vi "Register Assert.vi"(11 "Properties.Assert in":refnum<class "Properties.Assert.lvclass">) -> (3 "Properties.Assert out":refnum<class "Properties.Assert.lvclass">)   [LabVIEW 2013, in "Caraya.lvlib" / "Properties.Assert.lvclass"]
uses:
  Properties.Assert.lvclass
  Test Manager Message Assertion/TestManagerMsg.Assertion.lvclass
  Test Manager Message Assertion/Assert-Data -- cluster.ctl
  Properties.Assert.lvclass/Properties.Assert.ctl
  Properties/Properties.lvclass/Properties.ctl
  Properties/Properties.lvclass
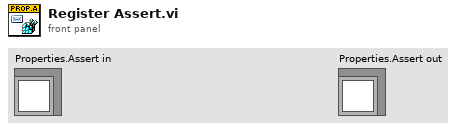
[diagram p1: front panel]
types:
  T1 = typedef "Caraya.lvlib/TestManagerMsg.Assertion.lvclass/Assert-Data -- cluster.ctl" = cluster{"Label":string, "Asserted":bool, "call-chain":string[], "upstream-error":errorcluster, "timestamp":timestamp, "Execution time (s)":dbl}
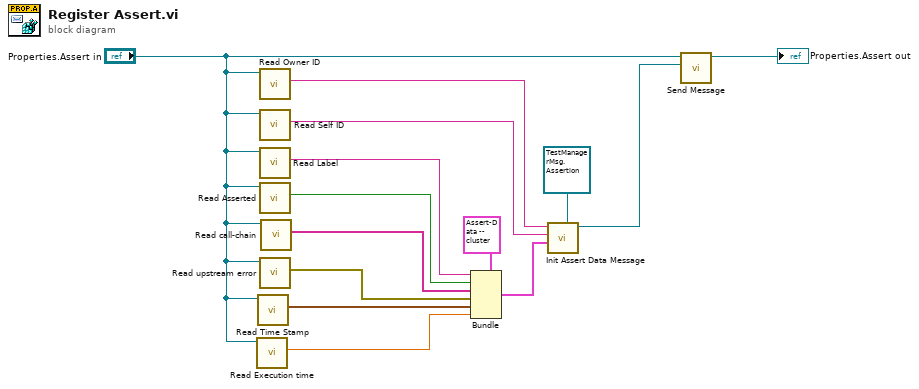
[diagram p0: block diagram]
diagram:
  n1 = call "Read Execution time.vi"("Properties.Assert in"="Properties.Assert in") -> ("Execution time (s)"=w5:dbl)  [unwired: 9 in, 1 out]
  n2 = call "Read Time Stamp.vi"("Properties in"="Properties.Assert in") -> ("Time Stamp"=w11:timestamp)  [unwired: 9 in, 1 out]
  n3 = call "Read Owner ID.vi"("Properties in"="Properties.Assert in") -> ("owner-id"=w2:string)  [unwired: 9 in, 1 out]
  n4 = call "Read Self ID.vi"("Properties in"="Properties.Assert in") -> ("self-id"=w3:string)  [unwired: 9 in, 1 out]
  n5 = call "Read Label.vi"("Properties in"="Properties.Assert in") -> ("Test Label"=w12:string)  [unwired: 9 in, 1 out]
  n6 = call "Read Asserted.vi"("Properties.Assert in"="Properties.Assert in") -> ("Asserted"=w9:bool)  [unwired: 9 in, 1 out]
  n7 = call "Read upstream error.vi"("Properties.Assert in"="Properties.Assert in") -> ("upstream-error"=w8:errorcluster)  [unwired: 9 in, 1 out]
  n8 = call "Read call-chain.vi"("Properties in"="Properties.Assert in") -> ("call-chain"=w10:string[])  [unwired: 9 in, 1 out]
  n9 = Bundle(cluster=T1 {"Label"="", "Asserted"=FALSE, "call-chain"=[], "upstream-error"={"status"=FALSE, "code"=0, "source"=""}, "timestamp"=timestamp(0 s since 1904-01-01), "Execution time (s)"=-1.0} ("Assert Data"), "Label"=w12, "Asserted"=w9, "call-chain"=w10, "upstream-error"=w8, "timestamp"=w11, "Execution time (s)"=w5) -> (w4:T1)
  n10 = call "Init Assert Data Message.vi"("Assert Data Message"=refnum<class "TestManagerMsg.Assertion.lvclass"> refnum ("Caraya.lvlib:TestManagerMsg.Assertion.lvclass"), "Assert Data"=w4, "AssertID"=w3, "TestID"=w2) -> ("Message"=w7:refnum<class "TestManagerMsg.lvclass">)  [unwired: 7 in]
  n11 = call "Send Message.vi"("TestManagerMsg"=w7, "Properties in"="Properties.Assert in") -> ("Properties out"=→"Properties.Assert out":refnum<class "Properties.Assert.lvclass">)  [unwired: 8 in, 1 out]
